vi "Fill dead ends.vi"(8 "error in (no error)":errorcluster, 11 "Maze in":refnum<class "Maze.lvclass">) -> (0 "error out":errorcluster, 3 "Maze out":refnum<class "Maze.lvclass">)   [LabVIEW 2021, in "Maze.lvclass"]
uses:
  Maze.lvclass
  Maze.lvclass/Maze.ctl
panel:
  out "size(s)":i32
  out "Numeric":i32
  out "Maze 2":string[][](array[string])
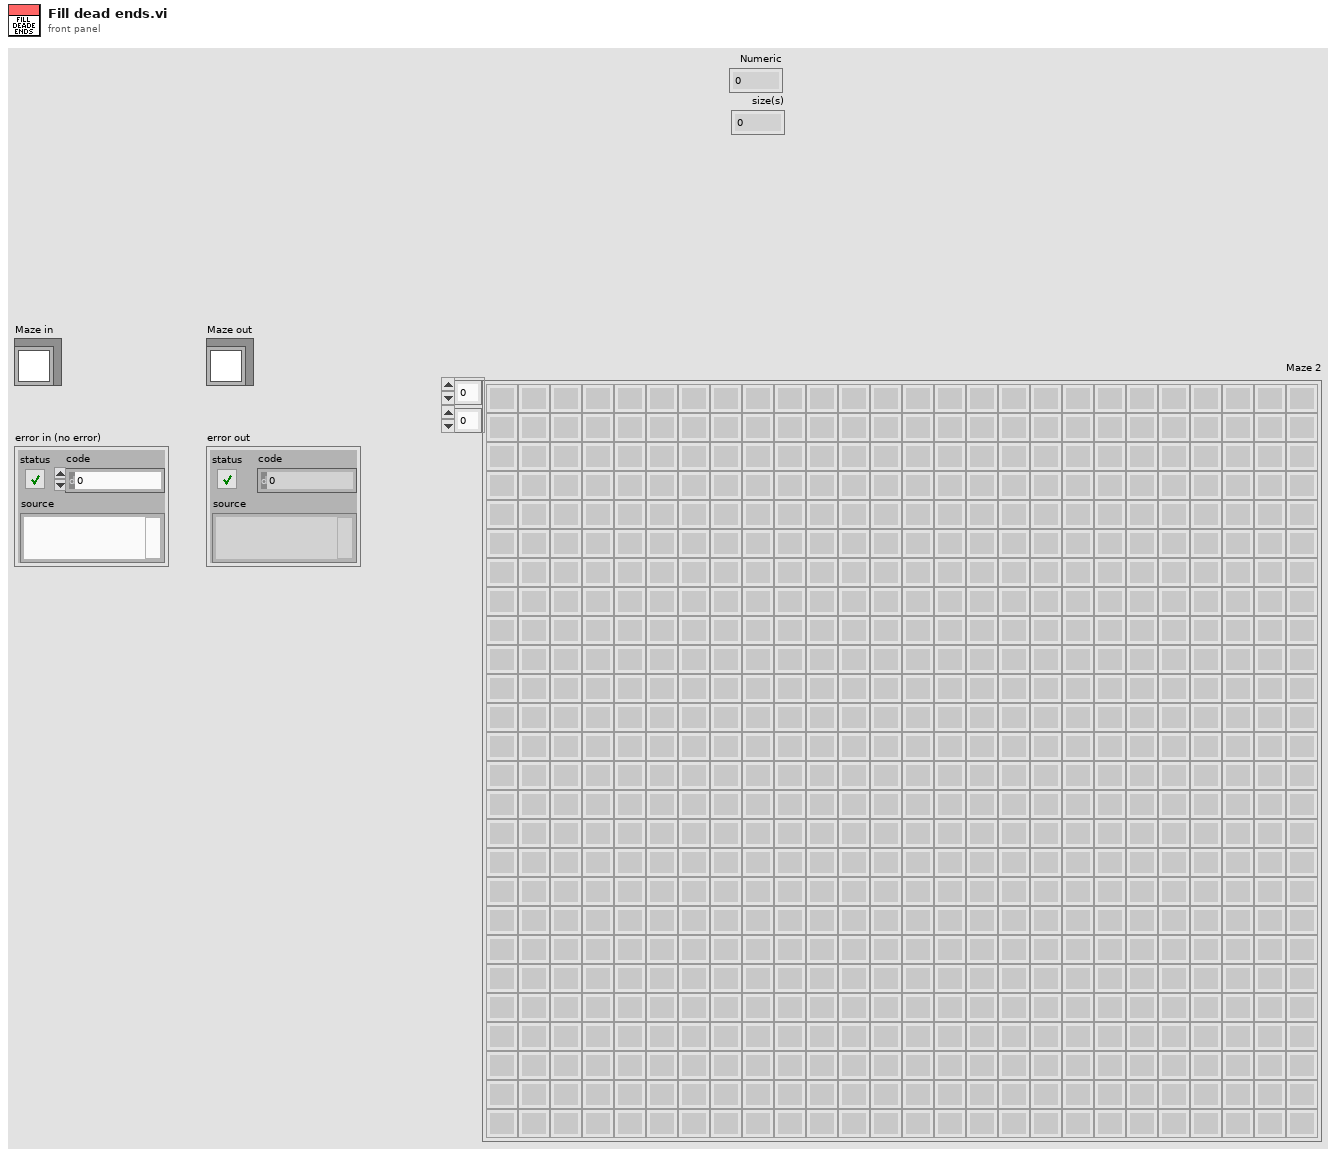
[diagram p1: front panel]
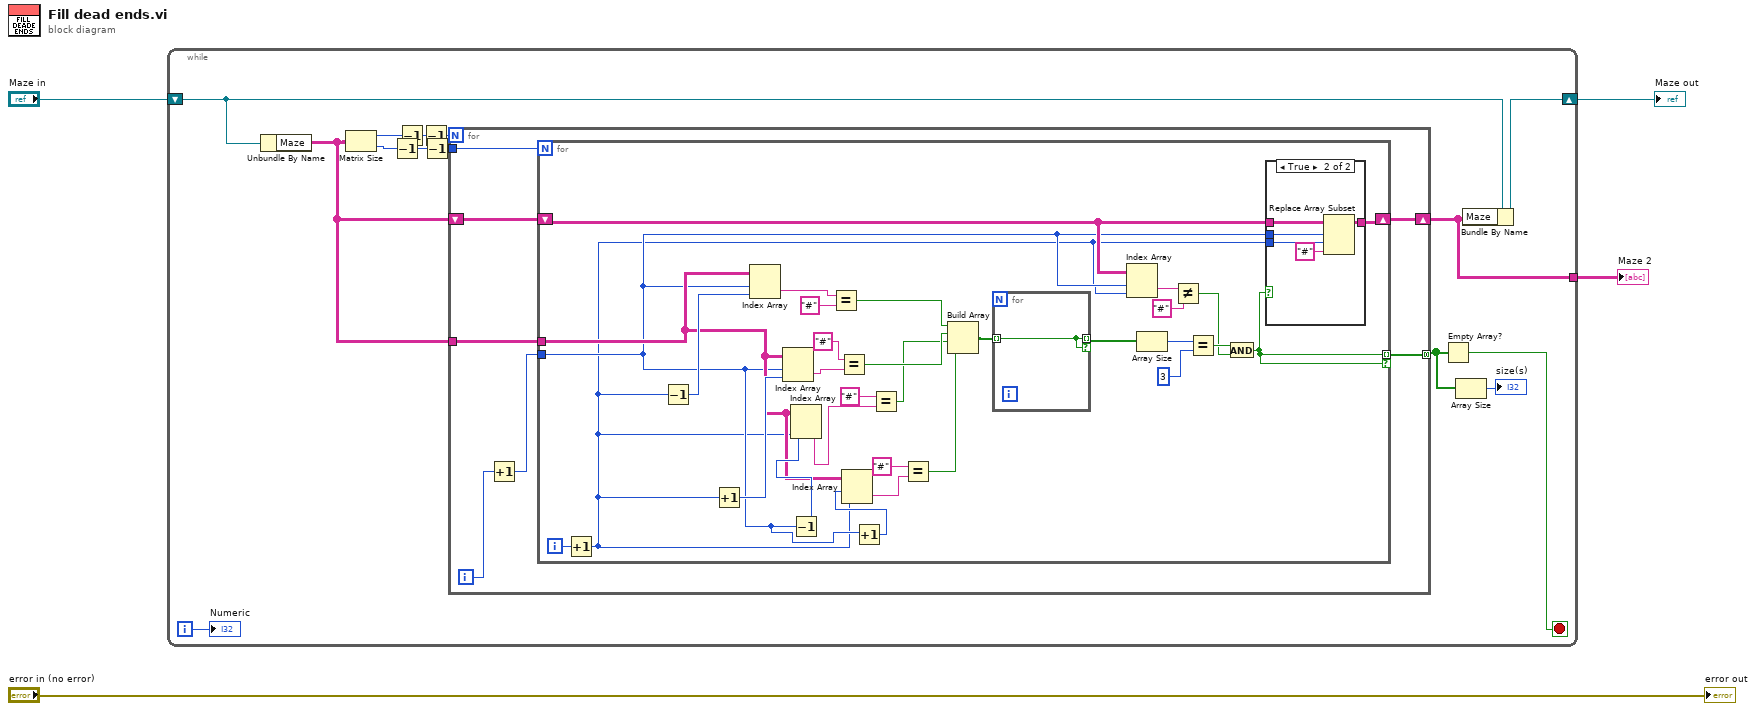
[diagram p0: block diagram]
diagram:
  n1 = while {
    shift-right: [w15] -> w2
    shift-left: "Maze in" -> [w18]
    tunnel: [w13] -> w1
    i -> [w12]
    stop <- w14 stop-if-true
    n2 = Unbundle By Name(w18) -> ("Maze"=w16:string[][])
    n3 = Matrix Size(0:w16) -> (1:w9:i32, 2:w17:i32)
    n4 = Decrement(x=w17) -> (x-1=w10:i32)
    n5 = Decrement(x=w9) -> (x-1=w8:i32)
    n6 = Decrement(x=w8) -> (x-1=w7:i32)
    n7 = Decrement(x=w10) -> (x-1=w11:i32)
    n8 = for {
      N: w7 -> [_]
      tunnel: w11 -> [w25]
      tunnel: w16 -> [w24]
      shift-right: [w21] -> w13
      shift-left: w16 -> [w23]
      tunnel: [w20] -> w6 mode=concatenating
      i -> [w22]
      n9 = Increment(x=w22) -> (x+1=w19:i32)
      n10 = for {
        N: w25 -> [_]
        tunnel: w24 -> [w53]
        shift-right: [w35] -> w21
        shift-left: w23 -> [w32]
        tunnel: w19 -> [w31]
        tunnel: [w27] -> w20 mode=indexing if=w27
        i -> [w34]
        n11 = Increment(x=w34) -> (x+1=w30:i32)
        n12 = Decrement(x=w30) -> (x-1=w56:i32)
        n13 = Increment(x=w30) -> (x+1=w55:i32)
        n14 = Index Array(array=w53, index (row)=w31, index (col)=w56) -> (element=w51:string)
        n15 = Index Array(array=w53, index (row)=w31, index (col)=w55) -> (element=w49:string)
        n16 = Decrement(x=w31) -> (x-1=w54:i32)
        n17 = Index Array(array=w53, index (row)=w54, index (col)=w30) -> (element=w47:string)
        n18 = Equal?(x=w51, y="#") -> (x = y?=w43:bool)
        n19 = Equal?(x="#" ("y"), y=w49) -> (x = y?=w42:bool)
        n20 = Increment(x=w31) -> (x+1=w52:i32)
        n21 = Index Array(array=w53, index (row)=w52, index (col)=w30) -> (element=w44:string)
        n22 = Equal?(x="#", y=w47) -> (x = y?=w41:bool)
        n23 = Equal?(x="#", y=w44) -> (x = y?=w40:bool)
        n24 = Build Array(w43, w42, w41, w40) -> (w39:bool[])
        n25 = for {
          tunnel: w39 -> [w63] mode=indexing
          tunnel: [w63] -> w38 mode=indexing if=w63
        }
        n26 = Index Array(array=w32, index (row)=w31, index (col)=w30) -> (element=w29:string)
        n27 = Array Size(array=w38) -> (size(s)=w37:i32)
        n28 = Not Equal?(x=w29, y="#" ("new element/subarray")) -> (x != y?=w26:bool)
        n29 = Equal?(x=w37, y=3) -> (x = y?=w33:bool)
        n30 = And(x=w33, y=w26) -> (x .and. y?=w27:bool)
        n31 = case shown="True" w27 {
          tunnel: [w57 w62] -> w35
          tunnel: w32 -> [w57 w61]
          tunnel: w31 -> [_ w60]
          tunnel: w30 -> [_ w59]
          frame False {
          }
          frame True {
            n32 = Replace Array Subset(array=w61, new element="#" ("new element/subarray"), index (row)=w60, index (col)=w59) -> (w62:string[][])
          }
        }
      }
    }
    n33 = Empty Array?(array=w6) -> (empty?=w14:bool)
    n34 = Array Size(array=w6) -> (size(s)=→"size(s)":i32)
    n35 = Bundle By Name(cluster=w18, "Maze"=w13) -> (w15:refnum<class "Maze.lvclass">)
    "Numeric" <- w12
  }
  "Maze out" <- w2
  "Maze 2" <- w1
  "error out" <- "error in (no error)"
